vi "Main.vi"() -> ()   [LabVIEW 2016]
uses:
  adsorbed_cluster.ctl
  auxiliary_cluster.ctl
  EOS.ctl
  pressure_cluster.ctl
panel:
  in  "File Name":string
  out "rho_bulk (g/cc)":dbl
  in  "Max Duration (hrs)":dbl(slide)=6.0 min=6.0 max=24.0 step=1.0 scale=6.0..24.0
  in  "Auxiliary Data":T1 {"EOS" items=["Ideal", "CH4_van_der_Waal", "CH4_Redlich_Kwong", "CO2_van_der_Waal", "CO2_Redlich_Kwong", ""]}
  out "z":dbl
  out "Vv (ml)":dbl
  out "P Chart":dbl(graph)
  in  "Stop Button":bool
  in  "Start Button":bool
  out "n Chart":T3(graph)
  out "Last Reading":T4 {"Pressure (barg)" scale=0.0..70.0}
  out "Duration (secs)":dbl(slide) scale=0.0..21600.0
  in  "Frequency (secs)":u32(slide)=10 min=1 max=600 step=1 scale=1.0..600.0
  # "Manometric Adsorption Measurement Rig"
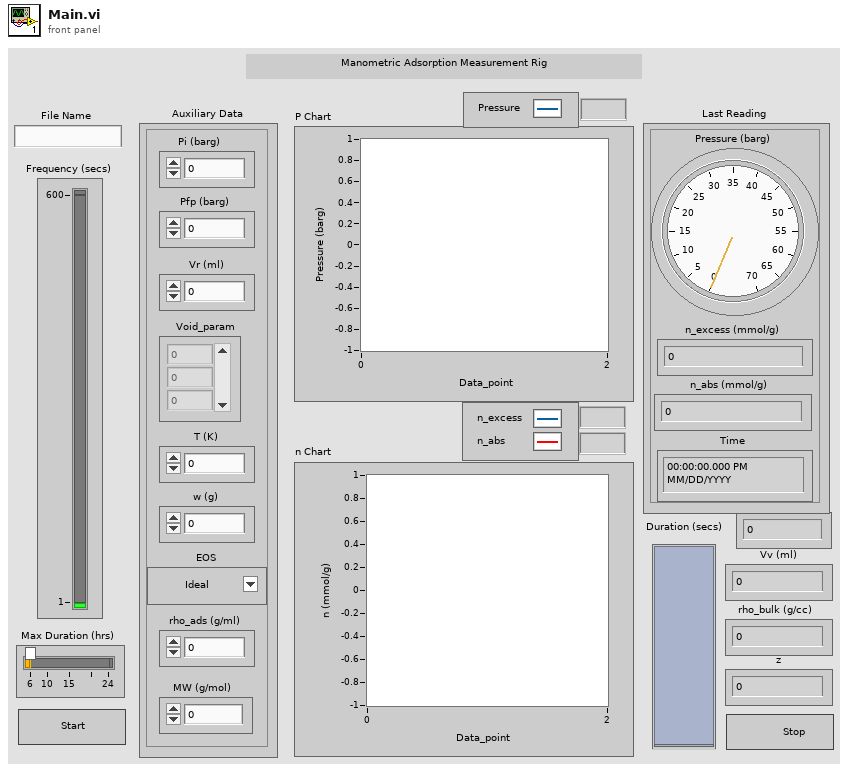
[diagram p1: front panel]
types:
  T1 = typedef "auxiliary_cluster.ctl" = cluster{"Pi (barg)":dbl, "Pfp (barg)":dbl, "Vr (ml)":dbl, "T (K)":dbl, "w (g)":dbl, "Void_param":dbl[], "EOS":T2, "rho_ads (g/ml)":dbl, "MW (g/mol)":dbl}
  T2 = typedef "EOS.ctl" = u16
  T3 = cluster{"n_excess (mmol/g)":dbl, "n_abs (mmol/g)":dbl}
  T4 = typedef "adsorbed_cluster.ctl" = cluster{"Time":timestamp, "Pressure (barg)":dbl, "n_excess (mmol/g)":dbl, "n_abs (mmol/g)":dbl}
  T5 = cluster{"n_excess (mmol/g)":dbl, "n_abs (mmol/g)":dbl}[]
  T6 = typedef "pressure_cluster.ctl" = cluster{"Time":timestamp, "Pressure (barg)":dbl}
  T7 = enum8{"Enabled", "Disabled", "Disabled and Grayed Out"}
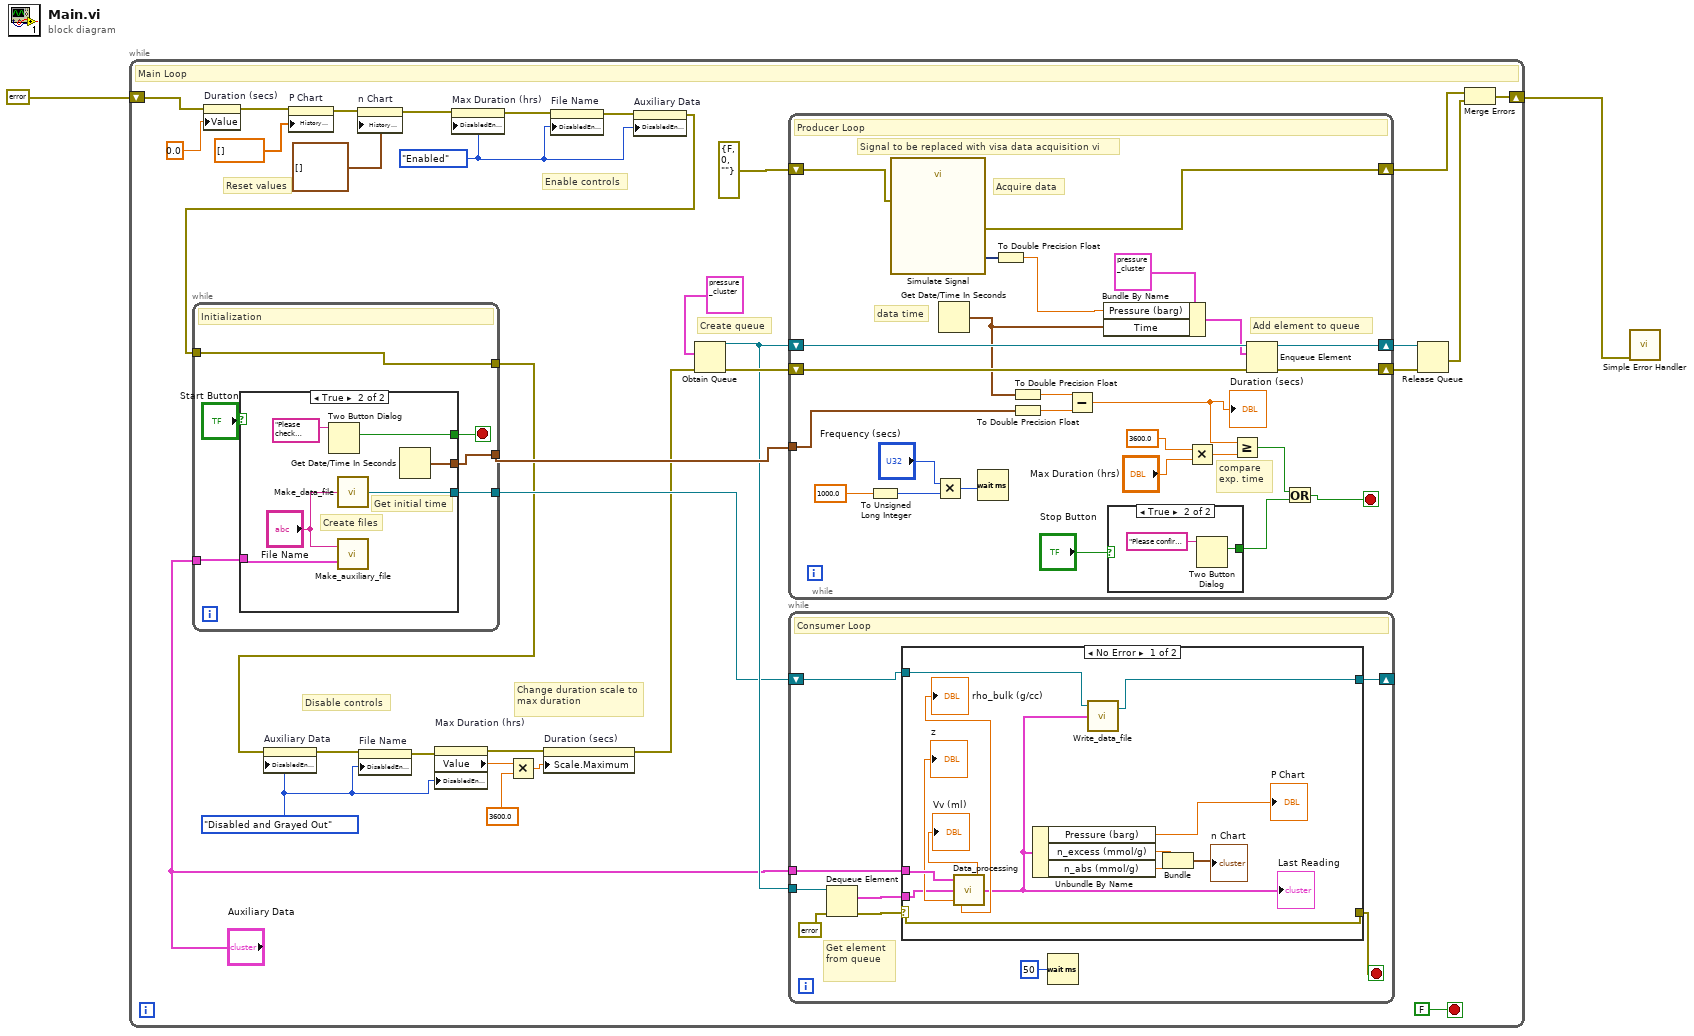
[diagram p0: block diagram]
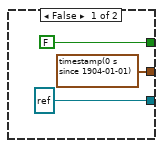
[diagram p2: hidden frame]
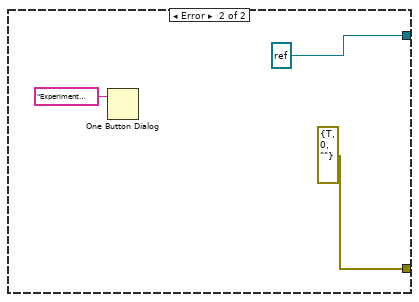
[diagram p3: hidden frame]
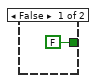
[diagram p4: hidden frame]
diagram:
  n1 = while {
    shift-right: [w26] -> w2
    shift-left: errorcluster {"status"=FALSE, "code"=0, "source"=""} ("error in (no error)") -> [w21]
    stop <- FALSE stop-if-true
    w7 = T7."Disabled and Grayed Out" ("Disabled")
    w11 = T7."Enabled" ("Disabled")
    # "Disable controls"
    # "Enable controls"
    # "Reset values"
    # "Create queue"
    # "Change duration scale to max duration"
    # "Main Loop"
    n2 = property on="Duration (secs)" class="Slide (strict)"(error in=w21, "Value"=0.0 ("Duration (hrs)")) -> (error out=w20:errorcluster)  [unwired: 1 in, 1 out]
    n3 = property on="P Chart" class="WFChart (strict)"(error in=w20, "History Data"=dbl[] []) -> (error out=w17:errorcluster)  [unwired: 1 in, 1 out]
    n4 = property on="n Chart" class="WFChart (strict)"(error in=w17, "History Data"=T5 []) -> (error out=w13:errorcluster)  [unwired: 1 in, 1 out]
    n5 = property on="Max Duration (hrs)" class="Slide (strict)"(error in=w13, "DisabledEnum"=w11) -> (error out=w12:errorcluster)  [unwired: 1 in, 1 out]
    n6 = property on="File Name" class="Str"(error in=w12, "DisabledEnum"=w11) -> (error out=w15:errorcluster)  [unwired: 1 in, 1 out]
    n7 = property on="Auxiliary Data" class="Clust (strict)"(error in=w15, "DisabledEnum"=w11) -> (error out=w14:errorcluster)  [unwired: 1 in, 1 out]
    n8 = while {
      tunnel: [w41] -> w10
      tunnel: w14 -> [w41]
      tunnel: [w36] -> w30
      tunnel: [w38] -> w25
      tunnel: "Auxiliary Data" -> [w37]
      stop <- w39 stop-if-true
      # "Initialization"
      n9 = case shown="True" "Start Button" {
        tunnel: [FALSE ("T button?") w50] -> w39
        tunnel: [refnum<file> refnum ("File Refnum") w47] -> w38
        tunnel: w37 -> [_ w46]
        tunnel: [timestamp(0 s since 1904-01-01) ("seconds since 1Jan1904") w45] -> w36
        frame False {
        }
        frame True {
          # "Get initial time"
          # "Create files"
          n10 = Two Button Dialog(message="Please check auxiliary data, file name, and max. duration and cofirm if you want to proceed.") -> (T button?=w50:bool)  [unwired: 2 in]
          n11 = call "Make_data_file.vi"("File Name"="File Name") -> ("File Refnum"=w47:refnum<file>)
          n12 = call "Make_auxiliary_file.vi"("Auxiliary Data"=w46, "File Name"="File Name") -> ()  [unwired: 1 out]
          n13 = Get Date/Time In Seconds() -> (seconds since 1Jan1904=w45:timestamp)
        }
      }
    }
    n14 = property on="Auxiliary Data" class="Clust (strict)"(error in=w10, "DisabledEnum"=w7) -> (error out=w9:errorcluster)  [unwired: 1 in, 1 out]
    n15 = property on="File Name" class="Str"(error in=w9, "DisabledEnum"=w7) -> (error out=w8:errorcluster)  [unwired: 1 in, 1 out]
    n16 = property on="Max Duration (hrs)" class="Slide (strict)"(error in=w8, "DisabledEnum"=w7) -> (error out=w23:errorcluster, "Value"=w4:dbl)  [unwired: 1 in, 1 out]
    n17 = Multiply(x=w4, y=3600.0) -> (x*y=w5:dbl)
    n18 = property on="Duration (secs)" class="Slide (strict)"(error in=w23, "Scale.Maximum"=w5) -> (error out=w6:errorcluster)  [unwired: 1 in, 1 out]
    n19 = Obtain Queue(element data type=T6 {"Time"=timestamp(0 s since 1904-01-01), "Pressure (barg)"=0.0} ("Presssure"), error in (no error)=w6) -> (queue out=w29:refnum<queue>, error out=w35:errorcluster)  [unwired: 3 in, 1 out]
    n20 = while {
      shift-right: [w93] -> w31
      shift-left: w29 -> [w94]
      shift-right: [w91] -> w32
      shift-left: w35 -> [w92]
      shift-right: [w99] -> w27
      shift-left: errorcluster {"status"=FALSE, "code"=0, "source"=""} ("error out") -> [w100]
      tunnel: w30 -> [w88]
      stop <- w86 stop-if-true
      # "Add element to queue"
      # "Acquire data"
      # "data time"
      # "compare exp. time"
      # "Signal to be replaced with visa data acquisition vi"
      # "Producer Loop"
      n21 = To Unsigned Long Integer(number=1000.0 ("y")) -> (unsigned 32bit integer=w95:u32)
      n22 = call "Simulate Signal"("error in (no error)"=w100) -> ("Triangle with Uniform Noise"=w101:dynamicdata, "error out"=w99:errorcluster)  [unwired: 13 in]
      n23 = Multiply(x="Frequency (secs)", y=w95) -> (x*y=w97:u32)
      n24 = Get Date/Time In Seconds() -> (seconds since 1Jan1904=w84:timestamp)
      n25 = Wait (ms)(milliseconds to wait=w97) -> ()  [unwired: 1 out]
      n26 = To Double Precision Float(number=w101) -> (double precision float=w82:dbl)
      n27 = To Double Precision Float(number=w84) -> (double precision float=w89:dbl)
      n28 = To Double Precision Float(number=w88) -> (double precision float=w90:dbl)
      n29 = Subtract(x=w89, y=w90) -> (x-y=w76:dbl)
      "Duration (secs)" <- w76
      n30 = Bundle By Name(cluster=T6 {"Time"=timestamp(0 s since 1904-01-01), "Pressure (barg)"=0.0} ("Presssure"), "Pressure (barg)"=w82, "Time"=w84) -> (w83:T6)
      n31 = case shown="True" "Stop Button" {
        tunnel: [FALSE ("T button?") w104] -> w81
        frame False {
        }
        frame True {
          n32 = Two Button Dialog(message="Please confirm if you want to stop the experiment, before max. duration.") -> (T button?=w104:bool)  [unwired: 2 in]
        }
      }
      n33 = Multiply(x=3600.0 ("y"), y="Max Duration (hrs)") -> (x*y=w77:dbl)
      n34 = Greater Or Equal?(x=w76, y=w77) -> (x >= y?=w87:bool)
      n35 = Enqueue Element(queue=w94, element=w83, error in (no error)=w92) -> (queue out=w93:refnum<queue>, error out=w91:errorcluster)  [unwired: 1 in, 1 out]
      n36 = Or(x=w87, y=w81) -> (x .or. y?=w86:bool)
    }
    n37 = while {
      tunnel: "Auxiliary Data" -> [w58]
      tunnel: w29 -> [w54]
      shift-right: [w51] -> _
      shift-left: w25 -> [w52]
      stop <- w59 stop-if-true
      # "Get element from queue"
      # "Consumer Loop"
      n38 = Dequeue Element(queue=w54, error in (no error)=errorcluster {"status"=FALSE, "code"=0, "source"=""}) -> (element=w56:T6, error out=w55:errorcluster)  [unwired: 1 in, 2 out]
      n39 = case shown="No Error" w55 {
        selector: w55 -> [w72 _]
        tunnel: w56 -> [w63 _]
        tunnel: [w72 errorcluster {"status"=TRUE, "code"=0, "source"=""} ("error IO")] -> w59
        tunnel: w58 -> [w70 _]
        tunnel: w52 -> [w62 _]
        tunnel: [w60 refnum<file> refnum ("output file refnum")] -> w51
        frame No Error {
          n40 = call "Data_processing.vi"("Presssure"=w63, "Auxiliary"=w70) -> ("z"=→"z":dbl, "Latest Data"=w61:T4, "V_v (ml)"=→"Vv (ml)":dbl, "rho_bulk"=→"rho_bulk (g/cc)":dbl)
          "Last Reading" <- w61
          n41 = Unbundle By Name(w61) -> ("Pressure (barg)"=→"P Chart":dbl, "n_excess (mmol/g)"=w66:dbl, "n_abs (mmol/g)"=w65:dbl)
          n42 = call "Write_data_file.vi"("Latest_Data"=w61, "Input file refnum"=w62) -> ("output file refnum"=w60:refnum<file>)  [unwired: 1 in, 1 out]
          n43 = Bundle("n_excess (mmol/g)"=w66, "n_abs (mmol/g)"=w65) -> (→"n Chart":T3)  [unwired: 1 in]
        }
        frame Error {
          n44 = One Button Dialog(message="Experiment complete.") -> ()  [unwired: 1 in, 1 out]
        }
      }
      n45 = Wait (ms)(milliseconds to wait=u32 50) -> ()  [unwired: 1 out]
    }
    n46 = Release Queue(queue=w31, error in (no error)=w32) -> (error out=w28:errorcluster)  [unwired: 1 in, 2 out]
    n47 = Merge Errors(w27, w28) -> (w26:errorcluster)
  }
  n48 = call <vilib>:"Simple Error Handler.vi"("error in (no error)"=w2) -> ()  [unwired: 4 in, 5 out]
